vi "MARS_Calculate_FoM.vi"(11 "Histogram":i32[](array[numeric])) -> (2 "FoM":dbl, 3 "Fit Histogram":i32[][](array[numeric]))   [LabVIEW 2015]
uses:
  MARS_Scan_Global_var.vi
  <vilib>/Analysis/NI_AAL_SigProc.lvlib
  <vilib>/Analysis/NI_AALPro.lvlib
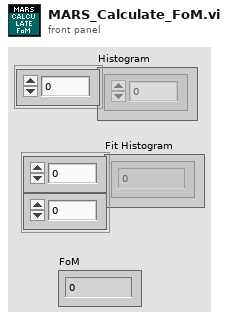
[diagram p1: front panel]
types:
  T1 = cluster{"initial amplitude":dbl, "initial center":dbl, "initial standard deviation":dbl, "offset":dbl}
  T2 = typedef "NI_AALPro.lvlib/Curve Fitting Criteria.ctl" = u16
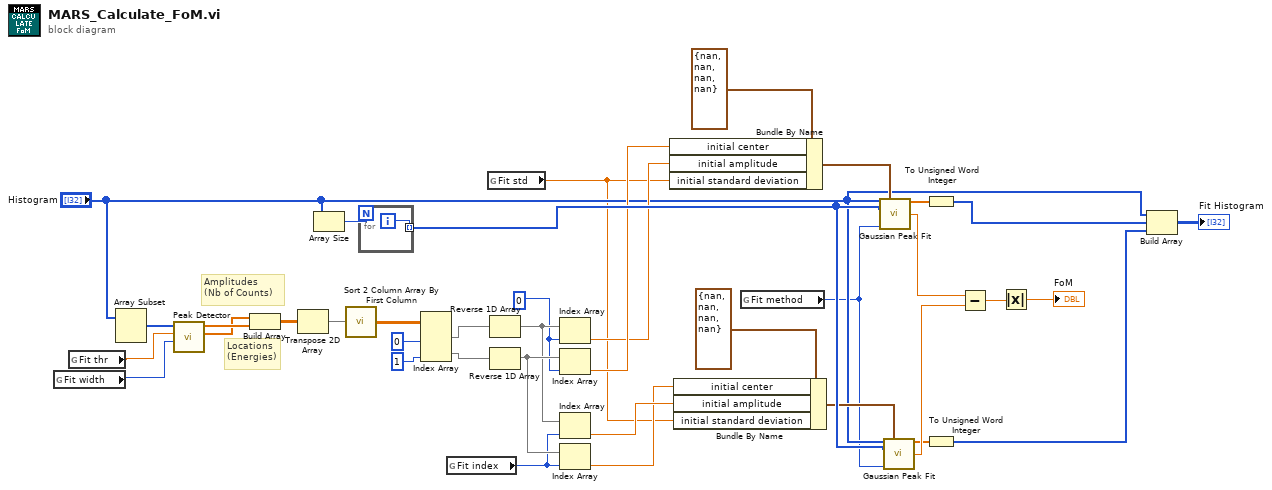
[diagram p0: block diagram]
diagram:
  w25 = 0 ("index")
  # "Locations\n(Energies)"
  # "Amplitudes\n(Nb of Counts)"
  n1 = global read "MARS_Scan_Global_var.vi" "Fit width"() -> (w4:i32)
  n2 = global read "MARS_Scan_Global_var.vi" "Fit thr"() -> (w5:dbl)
  n3 = Array Subset(array="Histogram") -> (w13:i32[])  [unwired: 2 in]
  n4 = call <vilib>:"Peak Detector.vi"("width"=w4, "threshold"=w5, "X"=w13) -> ("Amplitudes"=w21:dbl[], "Locations"=w22:dbl[])  [unwired: 4 in, 3 out]
  n5 = Build Array(w21, w22) -> (w14:dbl[][])
  n6 = Transpose 2D Array(2D array=w14) -> (transposed array=w15:dbl[][])
  n7 = Array Size(array="Histogram") -> (size(s)=w12:i32)
  n8 = call "Sort 2 Column Array By First Column.vi"("2D array to sort"=w15) -> ("Sorted array"=w16:dbl[][])
  n9 = for {
    N: w12 -> [_]
    tunnel: [w39] -> w32 mode=indexing
    i -> [w39]
  }
  n10 = Index Array(array=w16, index (col) #1=0 ("disabled index (col)"), index (col) #2=1 ("index (col)")) -> (element #1=w19:dbl[], element #2=w20:dbl[])  [unwired: 2 in]
  n11 = global read "MARS_Scan_Global_var.vi" "Fit index"() -> (w3:i32)
  n12 = global read "MARS_Scan_Global_var.vi" "Fit std"() -> (w2:dbl)
  n13 = Reverse 1D Array(array=w19) -> (reversed array=w26:dbl[])
  n14 = Reverse 1D Array(array=w20) -> (reversed array=w27:dbl[])
  n15 = Index Array(array=w26, index=w25) -> (element=w30:dbl)
  n16 = Index Array(array=w27, index=w25) -> (element=w31:dbl)
  n17 = Index Array(array=w26, index=w3) -> (element=w11:dbl)
  n18 = Index Array(array=w27, index=w3) -> (element=w10:dbl)
  n19 = Bundle By Name(cluster=T1 {"initial amplitude"=nan, "initial center"=nan, "initial standard deviation"=nan, "offset"=nan} ("initial guess"), "initial center"=w31, "initial amplitude"=w30, "initial standard deviation"=w2) -> (w24:T1)
  n20 = Bundle By Name(cluster=T1 {"initial amplitude"=nan, "initial center"=nan, "initial standard deviation"=nan, "offset"=nan} ("initial guess"), "initial center"=w10, "initial amplitude"=w11, "initial standard deviation"=w2) -> (w28:T1)
  n21 = global read "MARS_Scan_Global_var.vi" "Fit method"() -> (w1:T2)
  n22 = call <vilib>:"Gaussian Peak Fit.vi"("Y"="Histogram", "initial guess"=w24, "X"=w32, "method"=w1) -> ("Best Gaussian Fit"=w33:dbl[], "center"=w35:dbl)  [unwired: 5 in, 5 out]
  n23 = call <vilib>:"Gaussian Peak Fit.vi"("Y"="Histogram", "initial guess"=w28, "X"=w32, "method"=w1) -> ("Best Gaussian Fit"=w34:dbl[], "center"=w36:dbl)  [unwired: 5 in, 5 out]
  n24 = To Unsigned Word Integer(number=w33) -> (unsigned 16bit integer=w9:u16[])
  n25 = To Unsigned Word Integer(number=w34) -> (unsigned 16bit integer=w8:u16[])
  n26 = Subtract(x=w35, y=w36) -> (x-y=w37:dbl)
  n27 = Absolute Value(x=w37) -> (abs(x)=→"FoM":dbl)
  n28 = Build Array("Histogram", w9, w8) -> (→"Fit Histogram":i32[][])
